vi "Find_ballV2.vi"(0 "Image In":T1, 3 "error in":errorcluster) -> (4 "Image Out":T1, 5 "Plate coordinates":sgl[](array[numeric]), 6 "Ball Coordinates":cluster{"x":sgl, "y":sgl}, 7 "error out":errorcluster)   [LabVIEW 2021]
doc: "This VI extracts from an image the ball and plate coordinates. Plate coordinates are extracted with edge detection, then the coordinates of bottom left and top right points are reported. Ball coordinates are extracted using color matching from a test file"
uses:
  <vilib>/vision/Image Controls.llb/IMAQ Image.ctl
  <vilib>/vision/NI_Vision_Development_Module.lvlib
panel:
  in  "Camera Correction Path":path=path "C:/Users/EPFL/Documents/Vision/correction.png"
  in  "Test Ball Path":path=path "C:/Users/EPFL/Documents/Vision/test.png"
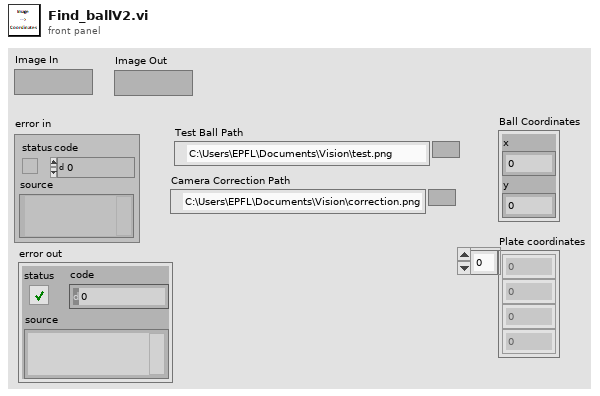
[diagram p1: front panel]
types:
  T1 = typedef "IMAQ Image.ctl" = refnum<image>
  T2 = cluster{"Feature":u32, "Points IDs":cluster{"GUID":string, "Index":i32}[]}[]
  T3 = typedef "Image Type" = u32
  T4 = cluster{"Global Rectangle":i32[], "Contours":cluster{"ID":enum32{"External", "Internal"}, "Type":u32, "Coordinates":i32[]}[]}
  T5 = cluster{"Show Search Area":bool, "Show Search Lines":bool, "Show Edges Found":bool, "Show Result":bool}
  T6 = cluster{"Number of Lines":i32, "Type":enum32{"First Edge Rake", "Best Edge Rake", "Hough Edge Rake", "First Edge Projection", "Best Edge Projection"}, "Min. Score":dbl, "Max. Score":dbl, "Orientation":dbl, "Angle Range":dbl, "Angle Tolerance":dbl, "Step Size":u32, "Min. SNR (db)":dbl, "Min. Points (%)":dbl, "Hough Iterations":i32}
  T7 = cluster{"Edge Polarity":u32, "Kernel Size":u32, "Width":u32, "Minimum Edge Strength":sgl, "Interpolation Type":enum32{"Zero Order", "Bilinear", "Quadratic", "Cubic", "Bilinear Fixed"}, "Data Processing Method":enum32{"Average", "Median"}}
  T8 = cluster{"Origin Pixel":cluster{"X":sgl, "Y":sgl}, "X Axis Pixel":cluster{"X":sgl, "Y":sgl}, "Axis Reference":u32}
  T9 = cluster{"Point1 (Pixels)":cluster{"X":sgl, "Y":sgl}, "Point2 (Pixels)":cluster{"X":sgl, "Y":sgl}, "Point1 (Real-World)":cluster{"X":sgl, "Y":sgl}, "Point2 (Real-World)":cluster{"X":sgl, "Y":sgl}, "Angle (Pixel)":dbl, "Angle (Real-World)":dbl, "Score":dbl, "Straightness":dbl, "Average SNR (db)":dbl, "Calibration Valid":bool}[]
  T10 = typedef "Search Line.ctl" = cluster{"Start Point":cluster{"X":sgl, "Y":sgl}, "End Point":cluster{"X":sgl, "Y":sgl}, "Edge Info":T11[], "Edge Map":dbl[], "Calibration Valid":bool}
  T11 = typedef "Edge New.ctl" = cluster{"Location (Pixel)":cluster{"X":sgl, "Y":sgl}, "Location (Real-World)":cluster{"X":sgl, "Y":sgl}, "Distance (Pixel)":dbl, "Distance (Real-World)":dbl, "Strength":dbl, "Noise":dbl, "Rising?":bool}
  T12 = cluster{"Straight Edges":cluster{"Point1 (Pixels)":cluster{"X":sgl, "Y":sgl}, "Point2 (Pixels)":cluster{"X":sgl, "Y":sgl}, "Point1 (Real-World)":cluster{"X":sgl, "Y":sgl}, "Point2 (Real-World)":cluster{"X":sgl, "Y":sgl}, "Angle (Pixel)":dbl, "Angle (Real-World)":dbl, "Score":dbl, "Straightness":dbl, "Average SNR (db)":dbl, "Calibration Valid":bool}[], "Search Lines Information":T10[], "Used Edges":cluster{"Edge Information":T11[]}[]}
  T13 = cluster{"Position":cluster{"x":sgl, "y":sgl}, "Angle":sgl, "Scale":sgl, "Score":sgl, "Bounding Box":cluster{"x":sgl, "y":sgl}[]}[]
  T14 = cluster{"Position":cluster{"x":sgl, "y":sgl}, "Angle":sgl, "Scale":sgl, "Score":sgl, "Bounding Box":cluster{"x":sgl, "y":sgl}[]}
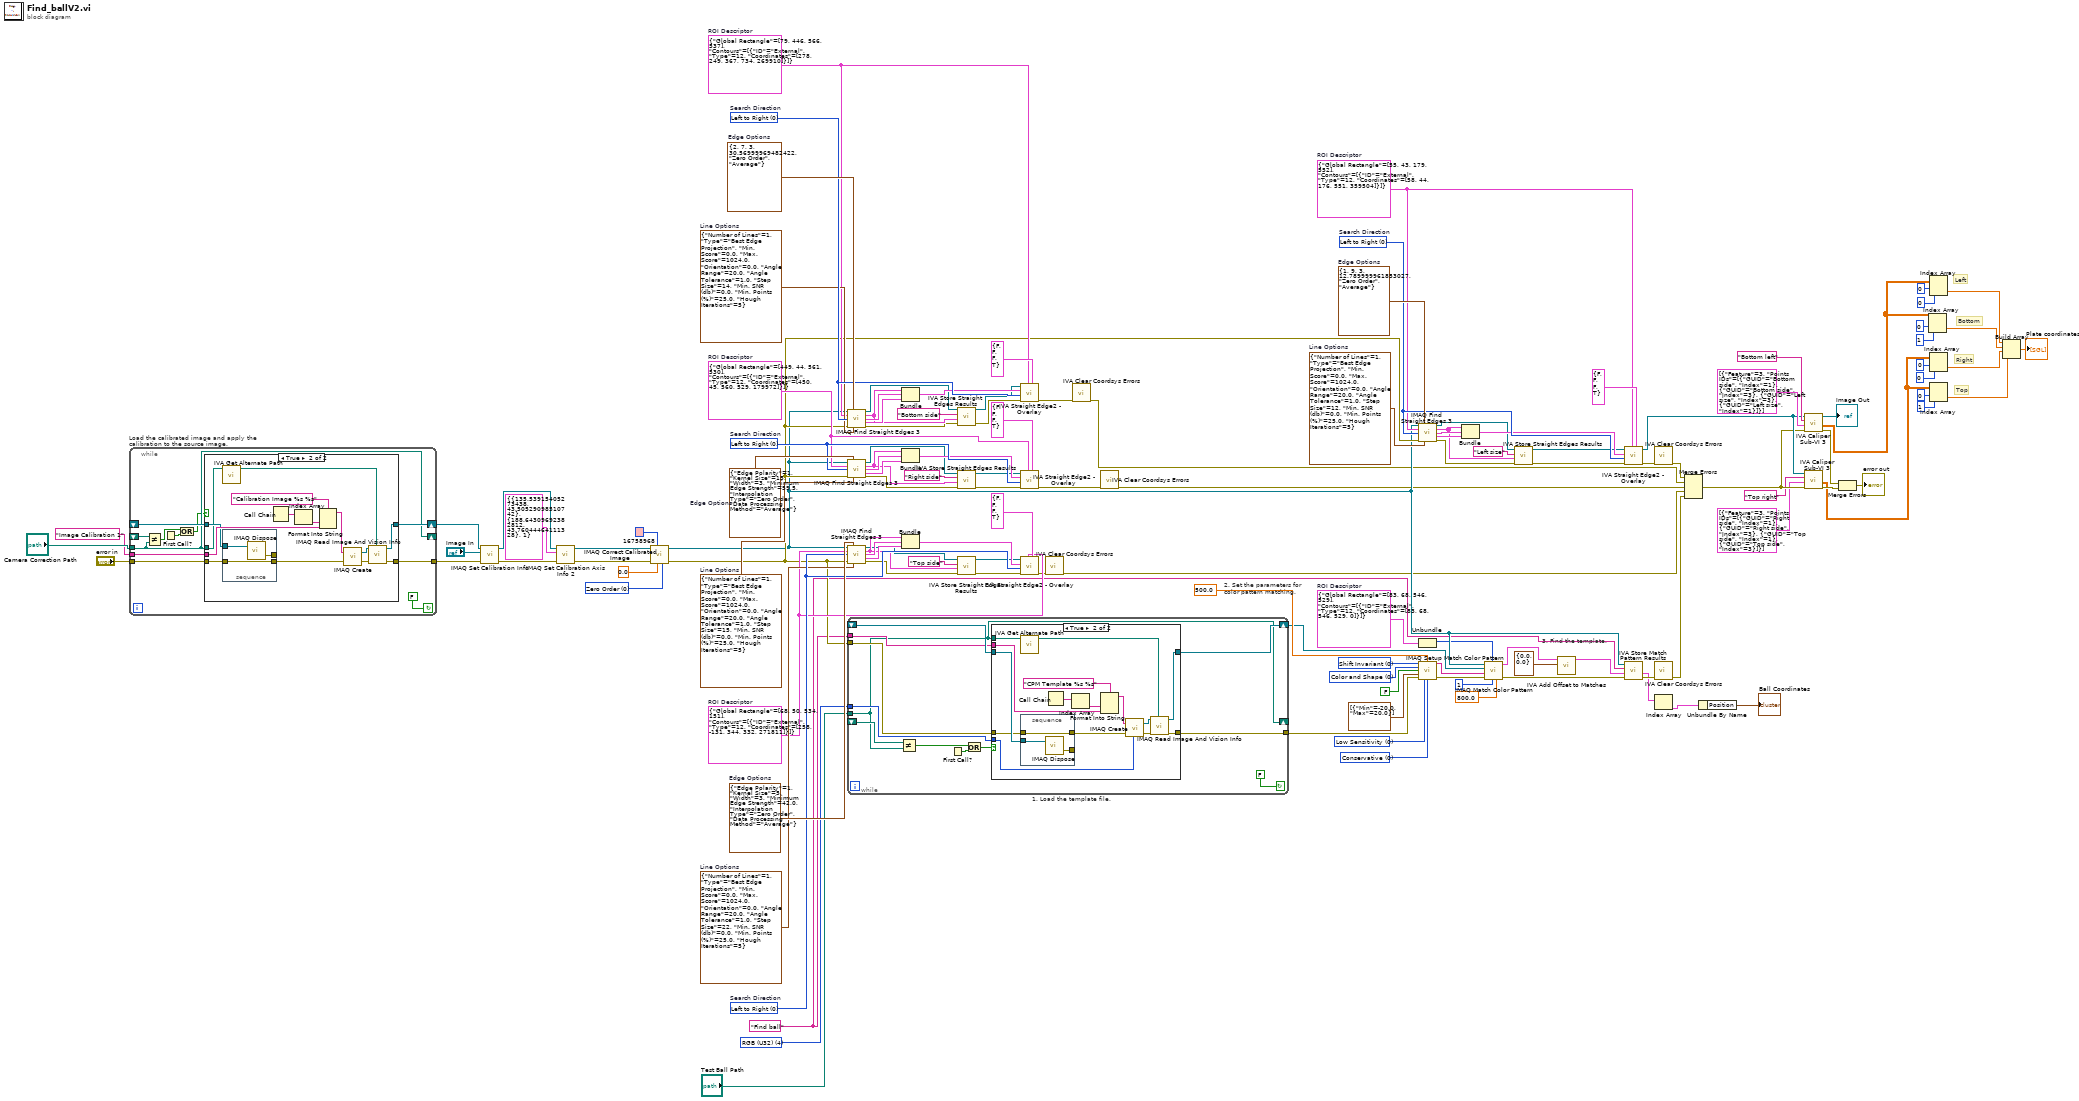
[diagram p0: block diagram]
diagram:
  w41 = "Find ball" ("Step Name")
  w49 = T3 4 items=["Grayscale (U8)", "Grayscale (I16)", "Grayscale (SGL)", "Complex (CSG)", "RGB (U32)", "HSL (U32)", "RGB (U64)"] ("Image Type")
  w52 = u32 0 items=["Conservative", "Balance", "Aggressive", "Very Aggressive"] ("Search Strategy")
  w53 = u32 0 items=["Low Sensitivity", "Medium Sensitivity", "High Sensitivity"] ("Color Sensitivity")
  w55 = u32 0 items=["Color and Shape", "Color", "Shape"] ("Match Feature Mode")
  w56 = u32 0 items=["Shift Invariant", "Rotation Invariant"] ("Match Mode")
  w46 = T4 {"Global Rectangle"=[83, 68, 546, 529], "Contours"=[{"ID"=enum."External", "Type"=12, "Coordinates"=[83, 68, 546, 529, 0]}]}  # ROI Descriptor
  w71 = T6 {"Number of Lines"=1, "Type"=enum."Best Edge Projection", "Min. Score"=0.0, "Max. Score"=1024.0, "Orientation"=0.0, "Angle Range"=20.0, "Angle Tolerance"=1.0, "Step Size"=22, "Min. SNR (db)"=0.0, "Min. Points (%)"=25.0, "Hough Iterations"=5}  # Line Options
  w72 = u32 0 items=["Left to Right", "Right to Left", "Top to Bottom", "Bottom to Top"]  # Search Direction
  w73 = T7 {"Edge Polarity"=1, "Kernel Size"=5, "Width"=3, "Minimum Edge Strength"=42.0, "Interpolation Type"=enum."Zero Order", "Data Processing Method"=enum."Average"}  # Edge Options
  w66 = T4 {"Global Rectangle"=[68, 50, 534, 151], "Contours"=[{"ID"=enum."External", "Type"=12, "Coordinates"=[258, -131, 344, 332, 271811]}]}  # ROI Descriptor
  w86 = T6 {"Number of Lines"=1, "Type"=enum."Best Edge Projection", "Min. Score"=0.0, "Max. Score"=1024.0, "Orientation"=0.0, "Angle Range"=20.0, "Angle Tolerance"=1.0, "Step Size"=15, "Min. SNR (db)"=0.0, "Min. Points (%)"=25.0, "Hough Iterations"=5}  # Line Options
  w87 = u32 0 items=["Left to Right", "Right to Left", "Top to Bottom", "Bottom to Top"]  # Search Direction
  w88 = T7 {"Edge Polarity"=1, "Kernel Size"=15, "Width"=3, "Minimum Edge Strength"=59.5, "Interpolation Type"=enum."Zero Order", "Data Processing Method"=enum."Average"}  # Edge Options
  w81 = T4 {"Global Rectangle"=[449, 44, 561, 530], "Contours"=[{"ID"=enum."External", "Type"=12, "Coordinates"=[450, 45, 560, 529, 179972]}]}  # ROI Descriptor
  w101 = T6 {"Number of Lines"=1, "Type"=enum."Best Edge Projection", "Min. Score"=0.0, "Max. Score"=1024.0, "Orientation"=0.0, "Angle Range"=20.0, "Angle Tolerance"=1.0, "Step Size"=14, "Min. SNR (db)"=0.0, "Min. Points (%)"=25.0, "Hough Iterations"=5}  # Line Options
  w102 = u32 0 items=["Left to Right", "Right to Left", "Top to Bottom", "Bottom to Top"]  # Search Direction
  w103 = T7 {"Edge Polarity"=2, "Kernel Size"=7, "Width"=3, "Minimum Edge Strength"=30.57, "Interpolation Type"=enum."Zero Order", "Data Processing Method"=enum."Average"}  # Edge Options
  w96 = T4 {"Global Rectangle"=[79, 446, 566, 537], "Contours"=[{"ID"=enum."External", "Type"=12, "Coordinates"=[278, 249, 367, 734, 269910]}]}  # ROI Descriptor
  w116 = T6 {"Number of Lines"=1, "Type"=enum."Best Edge Projection", "Min. Score"=0.0, "Max. Score"=1024.0, "Orientation"=0.0, "Angle Range"=20.0, "Angle Tolerance"=1.0, "Step Size"=12, "Min. SNR (db)"=0.0, "Min. Points (%)"=25.0, "Hough Iterations"=5}  # Line Options
  w117 = u32 0 items=["Left to Right", "Right to Left", "Top to Bottom", "Bottom to Top"]  # Search Direction
  w118 = T7 {"Edge Polarity"=1, "Kernel Size"=9, "Width"=3, "Minimum Edge Strength"=12.79, "Interpolation Type"=enum."Zero Order", "Data Processing Method"=enum."Average"}  # Edge Options
  w111 = T4 {"Global Rectangle"=[55, 43, 179, 552], "Contours"=[{"ID"=enum."External", "Type"=12, "Coordinates"=[58, 44, 176, 551, 359504]}]}  # ROI Descriptor
  w123 = u32 0 items=["Zero Order", "Bi-Linear", "Quadratic", "Cubic Spline"] ("Interpolation Type")
  # "Top"
  # "Right"
  # "Bottom"
  # "Left"
  # "2. Set the parameters for\ncolor pattern matching."
  # "3. Find the template."
  n1 = while "Load the calibrated image and apply the calibration to the source image." {
    shift-right: [w143] -> w130
    shift-left: _ -> [w142]
    tunnel: [w140] -> w129
    tunnel: "error in" -> [w139]
    tunnel: "Camera Correction Path" -> [w136]
    tunnel: "Image Calibration 1" ("Step Name") -> [w138]
    shift-right: [w136] -> _
    shift-left: _ -> [w137]
    stop <- FALSE continue-if-true
    n2 = Not Equal?(x=w137, y=w136) -> (x != y?=w134:bool)
    n3 = First Call?() -> (First Call?: T/F=w135:bool)
    n4 = Or(x=w134, y=w135) -> (x .or. y?=w133:bool)
    n5 = case shown="True" w133 {
      tunnel: [w145 w157] -> w143
      tunnel: w142 -> [w145 w149]
      tunnel: [w144 w154] -> w140
      tunnel: w139 -> [w144 w150]
      tunnel: w136 -> [_ w147]
      tunnel: w138 -> [_ w151]
      frame False {
      }
      frame True {
        n6 = call <vilib>:"IVA Get Alternate Path.vi"("Path In"=w147) -> ("Path Out"=w146:path)  [unwired: 10 out]
        n7 = stacked-sequence {
          tunnel: w150 -> [w161]
          tunnel: w149 -> [w162]
          tunnel: [w161] -> w148
          tunnel: [w160] -> _
          frame #0 {
            n8 = call "IMAQ Dispose"("Image"=w162) -> ("error out"=w160:errorcluster)  [unwired: 2 in, 3 out]
          }
        }
        n9 = Call Chain() -> (call chain=w153:string[])
        n10 = Index Array(array=w153) -> (element=w152:string)  [unwired: 1 in]
        n11 = Format Into String(format string="Calibration Image %s %s" ("Image Name"), w152, w151) -> (resulting string=w159:string)  [unwired: 2 in, 1 out]
        n12 = call "IMAQ Create"("Image Name"=w159, "error in (no error)"=w148) -> ("New Image"=w156:T1, "error out"=w155:errorcluster)  [unwired: 2 in, 1 out]
        n13 = call "IMAQ Read Image And Vision Info"("File Path"=w146, "error in (no error)"=w155, "Image"=w156) -> ("error out"=w154:errorcluster, "Image Out"=w157:T1)  [unwired: 1 in, 6 out]
      }
    }
  }
  n14 = call "IMAQ Set Calibration Info"("error in (no error)"=w129, "Image Dst"="Image In", "Image Src"=w130) -> ("error out"=w125:errorcluster, "Calibrated Image"=w126:T1)  [unwired: 1 in, 6 out]
  n15 = call-poly "IMAQ Set Calibration Axis Info 2"("error in (no error)"=w125, "Calibration Axis Info"=T8 {"Origin Pixel"={"X"=135.53915, "Y"=43.50529}, "X Axis Pixel"={"X"=188.6431, "Y"=43.760445}, "Axis Reference"=1}, "Calibration Template Image In"=w126) -> ("error out"=w121:errorcluster, "Calibration Template Image Out"=w122:T1)  [unwired: 7 out]
  n16 = call "IMAQ Correct Calibrated Image"("Interpolation Type"=w123, "Replace Value"=sgl 0.0, "Color Replace Value"=u32 16758968, "error in (no error)"=w121, "Image Src"=w122) -> ("error out"=w45:errorcluster, "Corrected Image"=w42:T1)  [unwired: 2 in, 3 out]
  n17 = call "IMAQ Find Straight Edges 3"("Image"=w42, "Edge Options"=w103, "ROI Descriptor"=w96, "Search Direction"=w102, "error in (no error)"=w45, "Line Options"=w101) -> ("Image (duplicate)"=w93:T1, "Straight Edges"=w94:T9, "Search Lines Information"=w98:T10[], "Used Edges"=w99:cluster{"Edge Information":T11[]}[], "error out"=w91:errorcluster)  [unwired: 1 in, 4 out]
  n18 = call "IMAQ Find Straight Edges 3"("Image"=w42, "Edge Options"=w88, "ROI Descriptor"=w81, "Search Direction"=w87, "error in (no error)"=w45, "Line Options"=w86) -> ("Image (duplicate)"=w78:T1, "Straight Edges"=w79:T9, "Search Lines Information"=w83:T10[], "Used Edges"=w84:cluster{"Edge Information":T11[]}[], "error out"=w76:errorcluster)  [unwired: 1 in, 4 out]
  n19 = call "IMAQ Find Straight Edges 3"("Image"=w42, "Edge Options"=w73, "ROI Descriptor"=w66, "Search Direction"=w72, "error in (no error)"=w45, "Line Options"=w71) -> ("Image (duplicate)"=w63:T1, "Straight Edges"=w64:T9, "Search Lines Information"=w68:T10[], "Used Edges"=w69:cluster{"Edge Information":T11[]}[], "error out"=w61:errorcluster)  [unwired: 1 in, 4 out]
  n20 = while "1. Load the template file." {
    shift-right: [w174] -> w36
    shift-left: _ -> [w173]
    tunnel: [w171] -> w35
    tunnel: w45 -> [w170]
    tunnel: "Test Ball Path" -> [w166]
    tunnel: w49 -> [w169]
    tunnel: w41 -> [w168]
    shift-right: [w166] -> _
    shift-left: _ -> [w167]
    stop <- FALSE continue-if-true
    n21 = Not Equal?(x=w167, y=w166) -> (x != y?=w164:bool)
    n22 = First Call?() -> (First Call?: T/F=w165:bool)
    n23 = Or(x=w164, y=w165) -> (x .or. y?=w163:bool)
    n24 = case shown="True" w163 {
      tunnel: [w176 w189] -> w174
      tunnel: w173 -> [w176 w181]
      tunnel: [w175 w186] -> w171
      tunnel: w170 -> [w175 w180]
      tunnel: w166 -> [_ w178]
      tunnel: w169 -> [_ w185]
      tunnel: w168 -> [_ w182]
      frame False {
      }
      frame True {
        n25 = call <vilib>:"IVA Get Alternate Path.vi"("Path In"=w178) -> ("Path Out"=w177:path)  [unwired: 10 out]
        n26 = stacked-sequence {
          tunnel: w181 -> [w194]
          tunnel: w180 -> [w193]
          tunnel: [w193] -> w179
          tunnel: [w192] -> _
          frame #0 {
            n27 = call "IMAQ Dispose"("Image"=w194) -> ("error out"=w192:errorcluster)  [unwired: 2 in, 3 out]
          }
        }
        n28 = Call Chain() -> (call chain=w184:string[])
        n29 = Index Array(array=w184) -> (element=w183:string)  [unwired: 1 in]
        n30 = Format Into String(format string="CPM Template %s %s" ("Image Name"), w183, w182) -> (resulting string=w191:string)  [unwired: 2 in, 1 out]
        n31 = call "IMAQ Create"("Image Name"=w191, "Image Type"=w185, "error in (no error)"=w179) -> ("New Image"=w188:T1, "error out"=w187:errorcluster)  [unwired: 1 in, 1 out]
        n32 = call "IMAQ Read Image And Vision Info"("File Path"=w177, "error in (no error)"=w187, "Image"=w188) -> ("error out"=w186:errorcluster, "Image Out"=w189:T1)  [unwired: 1 in, 6 out]
      }
    }
  }
  n33 = Bundle("Straight Edges"=w94, "Search Lines Information"=w98, "Used Edges"=w99) -> (w95:T12)  [unwired: 1 out]
  n34 = Bundle("Straight Edges"=w79, "Search Lines Information"=w83, "Used Edges"=w84) -> (w80:T12)  [unwired: 1 out]
  n35 = Bundle("Straight Edges"=w64, "Search Lines Information"=w68, "Used Edges"=w69) -> (w65:T12)  [unwired: 1 out]
  n36 = call <vilib>:"IVA Store Straight Edges Results.vi"("error in (no error)"=w91, "Straight Edges"=w94, "Step Name"="Bottom side", "Image in"=w93) -> ("error out"=w90:errorcluster, "Image dup"=w92:T1)  [unwired: 6 out]
  n37 = call <vilib>:"IVA Store Straight Edges Results.vi"("error in (no error)"=w76, "Straight Edges"=w79, "Step Name"="Right side", "Image in"=w78) -> ("error out"=w75:errorcluster, "Image dup"=w77:T1)  [unwired: 6 out]
  n38 = call <vilib>:"IVA Store Straight Edges Results.vi"("error in (no error)"=w61, "Straight Edges"=w64, "Step Name"="Top side", "Image in"=w63) -> ("error out"=w60:errorcluster, "Image dup"=w62:T1)  [unwired: 6 out]
  n39 = call <vilib>:"IVA Straight Edge2 - Overlay.vi"("Setup"=T5 {"Show Search Area"=FALSE, "Show Search Lines"=FALSE, "Show Edges Found"=FALSE, "Show Result"=TRUE}, "Search Area"=w96, "error in (no error)"=w90, "Scan Direction"=w102, "Edge Results"=w95, "Image In"=w92) -> ("error out"=w89:errorcluster)  [unwired: 1 in, 4 out]
  n40 = call <vilib>:"IVA Straight Edge2 - Overlay.vi"("Setup"=T5 {"Show Search Area"=FALSE, "Show Search Lines"=FALSE, "Show Edges Found"=FALSE, "Show Result"=TRUE}, "Search Area"=w81, "error in (no error)"=w75, "Scan Direction"=w87, "Edge Results"=w80, "Image In"=w77) -> ("error out"=w74:errorcluster)  [unwired: 1 in, 4 out]
  n41 = call <vilib>:"IVA Straight Edge2 - Overlay.vi"("Setup"=T5 {"Show Search Area"=FALSE, "Show Search Lines"=FALSE, "Show Edges Found"=FALSE, "Show Result"=TRUE}, "Search Area"=w66, "error in (no error)"=w60, "Scan Direction"=w72, "Edge Results"=w65, "Image In"=w62) -> ("error out"=w59:errorcluster)  [unwired: 1 in, 4 out]
  n42 = call <vilib>:"IVA Clear Coordsys Errors.vi"("error in (no error)"=w59) -> ("error out"=w30:errorcluster)  [unwired: 10 in]
  n43 = call <vilib>:"IVA Clear Coordsys Errors.vi"("error in (no error)"=w89) -> ("error out"=w32:errorcluster)  [unwired: 10 in]
  n44 = call <vilib>:"IVA Clear Coordsys Errors.vi"("error in (no error)"=w74) -> ("error out"=w31:errorcluster)  [unwired: 10 in]
  n45 = call "IMAQ Find Straight Edges 3"("Image"=w42, "Edge Options"=w118, "ROI Descriptor"=w111, "Search Direction"=w117, "error in (no error)"=w45, "Line Options"=w116) -> ("Image (duplicate)"=w108:T1, "Straight Edges"=w109:T9, "Search Lines Information"=w113:T10[], "Used Edges"=w114:cluster{"Edge Information":T11[]}[], "error out"=w106:errorcluster)  [unwired: 1 in, 4 out]
  n46 = Unbundle(w46) -> ("Global Rectangle"=w37:i32[])  [unwired: 1 out]
  n47 = call "IMAQ Setup Match Color Pattern"("Match Mode"=w56, "Color Score Weight"=sgl 500.0, "Match Feature Mode"=w55, "Subpixel Accuracy"=FALSE, "Rotation Angle Ranges (degrees)"=cluster{"Min":sgl, "Max":sgl}[] [{"Min"=-20.0, "Max"=20.0}], "error in (no error)"=w35, "Color Sensitivity"=w53, "Search Strategy"=w52) -> ("Match Color Pattern Setup Data"=w40:string, "error out"=w39:errorcluster)  [unwired: 1 in, 5 out]
  n48 = Bundle("Straight Edges"=w109, "Search Lines Information"=w113, "Used Edges"=w114) -> (w110:T12)  [unwired: 1 out]
  n49 = call "IMAQ Match Color Pattern"("Minimum Match Score"=sgl 800.0, "Number of Matches Requested"=1, "Optional Rectangle"=w37, "error in (no error)"=w39, "Match Color Pattern Setup Data"=w40, "Template Image"=w36, "Image"=w42) -> ("error out"=w43:errorcluster, "Matches"=w38:T13)  [unwired: 3 out]
  n50 = call <vilib>:"IVA Store Straight Edges Results.vi"("error in (no error)"=w106, "Straight Edges"=w109, "Step Name"="Left size", "Image in"=w108) -> ("error out"=w105:errorcluster, "Image dup"=w107:T1)  [unwired: 6 out]
  n51 = call <vilib>:"IVA Add Offset to Matches.vi"("Match Offset"=cluster{"X":sgl, "Y":sgl} {"X"=0.0, "Y"=0.0}, "Matches in"=w38) -> ("Matches out"=w44:T13)  [unwired: 9 out]
  n52 = call <vilib>:"IVA Straight Edge2 - Overlay.vi"("Setup"=T5 {"Show Search Area"=FALSE, "Show Search Lines"=FALSE, "Show Edges Found"=FALSE, "Show Result"=TRUE}, "Search Area"=w111, "error in (no error)"=w105, "Scan Direction"=w117, "Edge Results"=w110, "Image In"=w107) -> ("error out"=w104:errorcluster, "Image Out"=w26:T1)  [unwired: 1 in, 3 out]
  n53 = call <vilib>:"IVA Store Match Pattern Results.vi"("error in (no error)"=w43, "Matches"=w44, "Step Name"=w41, "Image in"=w42) -> ("error out"=w34:errorcluster, "Calibrated Matches"=w1:T13)  [unwired: 6 out]
  n54 = call <vilib>:"IVA Clear Coordsys Errors.vi"("error in (no error)"=w104) -> ("error out"=w33:errorcluster)  [unwired: 10 in]
  n55 = call <vilib>:"IVA Clear Coordsys Errors.vi"("error in (no error)"=w34) -> ("error out"=w29:errorcluster)  [unwired: 10 in]
  n56 = Index Array(array=w1) -> (element=w2:T14)  [unwired: 1 in]
  n57 = Merge Errors(w33, w32, w31, w30, w29) -> (w25:errorcluster)
  n58 = Unbundle By Name(w2) -> ("Position"=→"Ball Coordinates":cluster{"x":sgl, "y":sgl})
  n59 = call <vilib>:"IVA Caliper Sub-VI 3.vi"("error in"=w25, "Parameters"=T2 [{"Feature"=3, "Points IDs"=[{"GUID"="Bottom side", "Index"=1}, {"GUID"="Bottom side", "Index"=3}, {"GUID"="Left size", "Index"=3}, {"GUID"="Left size", "Index"=1}]}], "Step Name"="Bottom left", "Image In"=w26) -> ("error out"=w20:errorcluster, "Results (Calibrated)"=w5:sgl[][], "Image Out"=→"Image Out":T1)  [unwired: 1 in, 4 out]
  n60 = call <vilib>:"IVA Caliper Sub-VI 3.vi"("error in"=w25, "Parameters"=T2 [{"Feature"=3, "Points IDs"=[{"GUID"="Right side", "Index"=1}, {"GUID"="Right side", "Index"=3}, {"GUID"="Top side", "Index"=1}, {"GUID"="Top side", "Index"=3}]}], "Step Name"="Top right", "Image In"=w26) -> ("error out"=w19:errorcluster, "Results (Calibrated)"=w4:sgl[][])  [unwired: 1 in, 5 out]
  n61 = Merge Errors(w20, w19) -> (→"error out":errorcluster)
  n62 = Index Array(array=w5, index (row)=0, index (col)=1 ("disabled index (col)")) -> (element=w13:sgl)
  n63 = Index Array(array=w4, index (row)=0, index (col)=0 ("disabled index (col)")) -> (element=w8:sgl)
  n64 = Index Array(array=w5, index (row)=0, index (col)=0 ("disabled index (col)")) -> (element=w14:sgl)
  n65 = Index Array(array=w4, index (row)=0, index (col)=1 ("disabled index (col)")) -> (element=w7:sgl)
  n66 = Build Array(w14, w13, w8, w7) -> (→"Plate coordinates":sgl[])
